vi "RT_Aerodynamic_Moment_in_DLR_Navigation_Reference_System_2 (SubVI).vi"(8 "input cluster":T2, 9 "Rotation":T1, 10 "i":i32, 11 "Data":dbl[][](array[numeric])) -> (3 "MFA (Nm)":dbl[](array[numeric]))   [LabVIEW 2017]
uses:
  <vilib>/Analysis/baseanly.llb/Real A x B.vi
  <vilib>/Analysis/Matrix/Numeric/Conversions/Array To Matrix - RA.vi
  <vilib>/Analysis/Matrix/Numeric/Conversions/Array To Matrix - RA2.vi
  <vilib>/Analysis/Matrix/Numeric/Conversions/Matrix To Array - RM.vi
  <vilib>/Analysis/NI_AALBase.lvlib
  <vilib>/Analysis/Matrix/NI_Matrix.lvlib
  <vilib>/Analysis/NI_AALPro.lvlib
panel:
  out "CoP (m)":dbl
  out "Ra":dbl[](array[numeric])
  out "ra":dbl
  out "CoG (m)":dbl
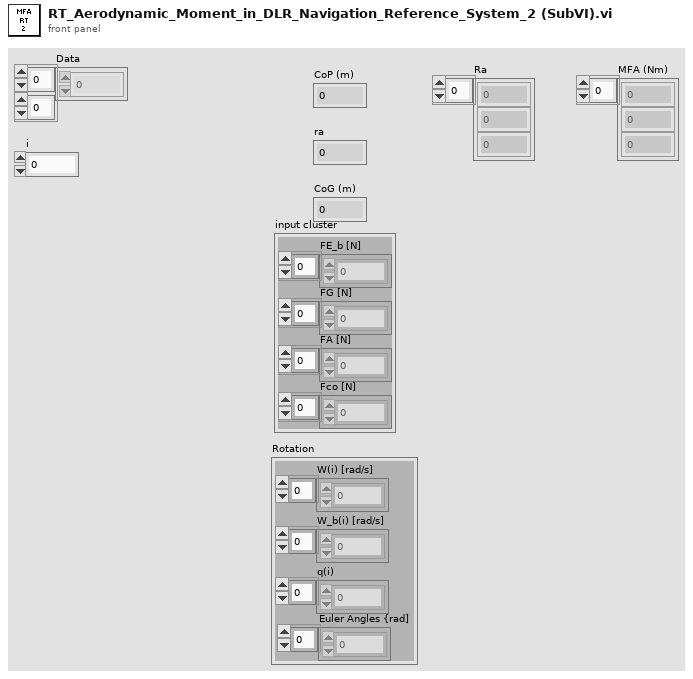
[diagram p1: front panel]
types:
  T1 = cluster{"W(i) [rad/s]":dbl[], "W_b(i) [rad/s]":dbl[], "q(i)":dbl[], "Euler Angles {rad]":dbl[]}
  T2 = cluster{"FE_b [N]":dbl[], "FG [N]":dbl[], "FA [N]":dbl[], "Fco [N]":dbl[]}
  T3 = typedef "NI_Matrix.lvlib/RealMatrix.ctl" = dbl[][]
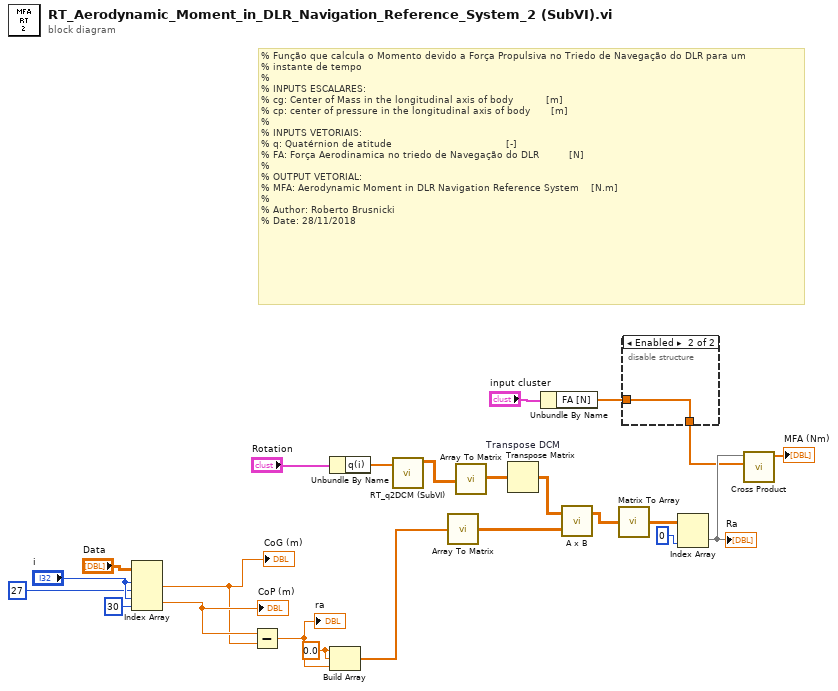
[diagram p0: block diagram]
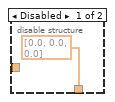
[diagram p2: hidden frame]
diagram:
  w14 = 0.0 ("element")
  # "% Função que calcula o Momento devido a Força Propulsiva no Triedo de Navegação do DLR para um \n% instante de tempo\n%\n% INPUTS ESCALARES:\n% cg: Center of Mass in the longitudinal axis of body           [m]\n% cp: center of pressure in the longitudinal axis of body       [m]\n% \n% INPUTS VETORIAIS:\n% q: Quatérnion de atitude                                      [-]\n% FA: Força Aerodinamica no triedo de Navegação do DLR          [N] \t\n%\n% OUTPUT VETORIAL:\n% MFA: Aerodynamic Moment in DLR Navigation Reference System    [N.m]\n%\n% Author: Roberto Brusnicki\n% Date: 28/11/2018"
  n1 = Index Array(array="Data", index (row) #1="i", index (col) #1=27 ("disabled index (col)"), index (row) #2="i", index (col) #2=30 ("disabled index (col)")) -> (element #1=w10:dbl, element #2=w23:dbl)
  "CoG (m)" <- w10
  "CoP (m)" <- w23
  n2 = Subtract(x=w23, y=w10) -> (x-y=w15:dbl)
  "ra" <- w15
  n3 = Unbundle By Name("Rotation") -> ("q(i)"=w4:dbl[])
  n4 = Build Array(w14, w14, w15) -> (w13:dbl[])
  n5 = call "RT_q2DCM (SubVI).vi"("Quaternion"=w4) -> ("DCM"=w3:dbl[][])  [unwired: 10 in]
  n6 = call-poly <vilib>:"Array To Matrix.vi"("Real 1D Array"=w13) -> ("Real Matrix (Column Vector)"=w16:T3)
  n7 = call-poly <vilib>:"Array To Matrix.vi"("Real 2D Array"=w3) -> ("Real Matrix"=w12:T3)
  n8 = Transpose Matrix "Transpose DCM"(1:w12) -> (0:w11:T3)
  n9 = Unbundle By Name("input cluster") -> ("FA [N]"=w6:dbl[])
  n10 = call-poly <vilib>:"A x B.vi"("B"=w16, "A"=w11) -> ("A x B"=w18:T3)  [unwired: 1 out]
  n11 = call-poly <vilib>:"Matrix To Array.vi"("Real Matrix"=w18) -> ("Real 2D Array"=w17:dbl[][])
  n12 = disable-structure shown="Enabled" {
    disable-tunnel: w6 -> [_ w25]
    disable-tunnel: [dbl[] [0.0, 0.0, 0.0] ("FA [N]") w25] -> w1
    frame Disabled {
    }
    frame Enabled {
    }
  }
  n13 = Index Array(array=w17, index (col)=0 ("index (row)")) -> (element=w9:dbl[])  [unwired: 1 in]
  "Ra" <- w9
  n14 = call <vilib>:"Cross Product.vi"("B Vector"=w1, "A Vector"=w9) -> ("Cross Product"=→"MFA (Nm)":dbl[])  [unwired: 8 in, 1 out]
